vi "ChangePanel.vi"(8 "error in (no error)":errorcluster, 9 "New Active Index":i32, 10 "Panel Index":i32, 11 "MAUI in":refnum<class "MAUI.lvclass">) -> (0 "error out":errorcluster, 3 "MAUI out":refnum<class "MAUI.lvclass">)   [LabVIEW 2019, in "MAUI.lvclass"]
doc: "This is responsible for changing panels. This is usually called when the user is trying to change the subpanel. Fairly straight forward."
uses:
  MAUI.lvclass
  MAUI.lvclass/MAUI.ctl
  <userlib>/LevyLab/Embedded UI/SMO.UI.Embedded/Embedded UI.lvclass
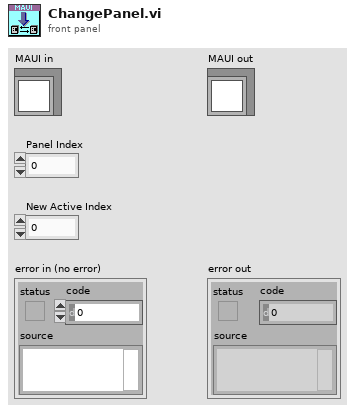
[diagram p1: front panel]
types:
  T1 = typedef "MAUI.lvclass/PanelData.ctl" = cluster{"SubPanel":refnum<vi>, "Ring":refnum<vi>, "Active":i32}
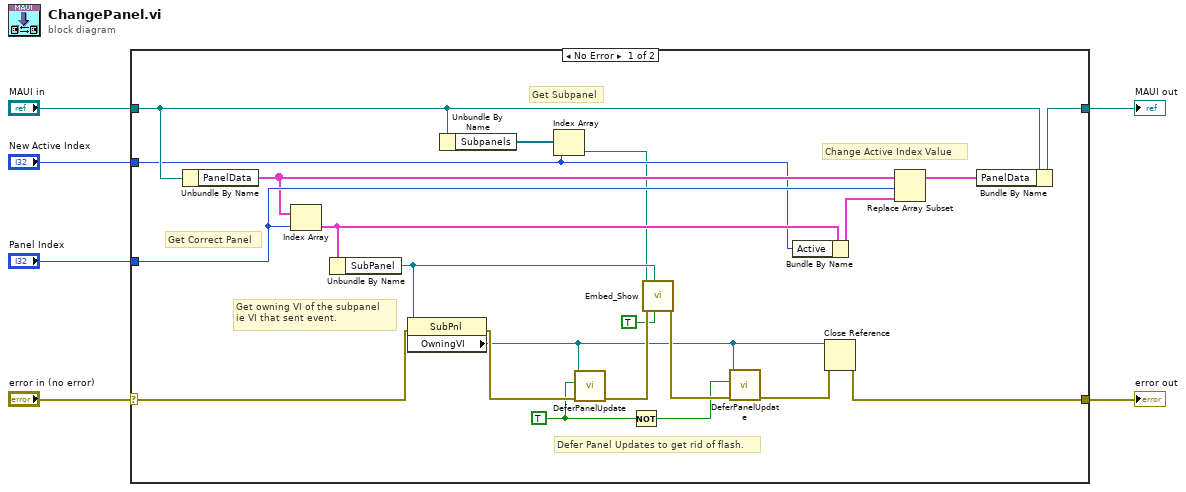
[diagram p0: block diagram]
diagram:
  n1 = case shown="No Error" "error in (no error)" {
    selector: "error in (no error)" -> [w27 w29]
    tunnel: [w26 w29] -> w5
    tunnel: [w16 w28] -> w3
    tunnel: "MAUI in" -> [w17 w28]
    tunnel: "Panel Index" -> [w18 _]
    tunnel: "New Active Index" -> [w13 _]
    frame No Error {
      w9 = TRUE
      # "Defer Panel Updates to get rid of flash."
      # "Get owning VI of the subpanel\nie VI that sent event."
      # "Get Subpanel"
      # "Change Active Index Value"
      # "Get Correct Panel"
      n2 = Unbundle By Name(w17) -> ("PanelData"=w15:T1[])
      n3 = Index Array(array=w15, index=w18) -> (element=w20:T1)
      n4 = Unbundle By Name(w20) -> ("SubPanel"=w12:refnum<vi>)
      n5 = property on="Property Node" class="SubPnl"(reference=w12, error in=w27) -> (error out=w25:errorcluster, "OwningVI"=w7:refnum<vi>)  [unwired: 1 out]
      n6 = Unbundle By Name(w17) -> ("Subpanels"=w21:refnum<class "Embedded UI.lvclass">[])
      n7 = Index Array(array=w21, index=w13) -> (element=w11:refnum<class "Embedded UI.lvclass">)
      n8 = call <userlib>:"DeferPanelUpdate.vi"("error in (no error)"=w25, "Defer Panel Updates"=w9, "VI in"=w7) -> ("error out"=w24:errorcluster)  [unwired: 8 in]
      n9 = Not(x=w9) -> (.not. x?=w8:bool)
      n10 = call <userlib>:"Embed_Show.vi"("Force?"=TRUE, "Sub Panel"=w12, "error in (no error)"=w24, "EmbeddedSMO in"=w11) -> ("error out"=w23:errorcluster)  [unwired: 6 in, 1 out]
      n11 = call <userlib>:"DeferPanelUpdate.vi"("error in (no error)"=w23, "Defer Panel Updates"=w8, "VI in"=w7) -> ("error out"=w22:errorcluster)  [unwired: 8 in]
      n12 = Bundle By Name(cluster=w20, "Active"=w13) -> (w19:T1)
      n13 = Close Reference(reference=w7, error in (no error)=w22) -> (error out=w26:errorcluster)
      n14 = Replace Array Subset(array=w15, new element=w19, index=w18) -> (w14:T1[])
      n15 = Bundle By Name(cluster=w17, "PanelData"=w14) -> (w16:refnum<class "MAUI.lvclass">)
    }
    frame Error {
    }
  }
  "error out" <- w5
  "MAUI out" <- w3
